vi "Array Of Variants To Class Types.vi"(7 "Elements":variant[](array[variant]), 8 "error in (no error)":errorcluster, 10 "Class types":variant[](array[variant]), 11 "Registry Variant Accessor in":refnum<class "CConfig Variant Accessor.lvclass">) -> (0 "error out":errorcluster, 2 "Class types":variant[](array[variant]), 3 "Registry Variant Accessor out":refnum<class "CConfig Variant Accessor.lvclass">)   [LabVIEW 2013, in "CConfig Variant Accessor.lvclass"]
doc: "Copyright 2018, Carya Automatisering, Wiebe Walstra."
uses:
  CConfig Variant Accessor.lvclass
  <vilib>/Utility/VariantDataType/Type.ctl
  <vilib>/Utility/VariantDataType/VariantType.lvlib
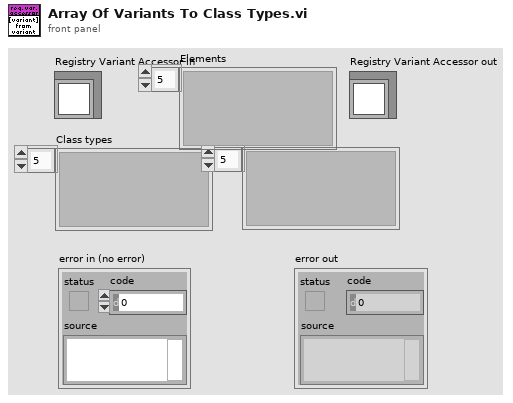
[diagram p1: front panel]
types:
  T1 = typedef "VariantType.lvlib/Type.ctl" = enum8{"Invalid Type", "Void", "I8", "I16", "I32", "I64", "U8", "U16", "U32", "U64", "Single Float", "Double Float", "Extended Float", "Single Complex", "Double Complex", "Extended Complex", "Enum U8", "Enum U16", "Enum U32", "Enum U64", "Single Float With Unit", "Double Float With Unit", "Extended Float With Unit", "Single Complex with Unit", "Double Complex with Unit", "Extended Complex with Unit", "Boolean", "String", "Path", "Picture", "Tag", "Array", "Cluster", "Variant", "LV Variant", "Waveform", "Timestamp", "Digital Waveform", "Digital Data", "ExpressData", "Refnum", "External Data", "VI", "Poly VI", "LabVIEW Class Instance", "Fixed Point"}
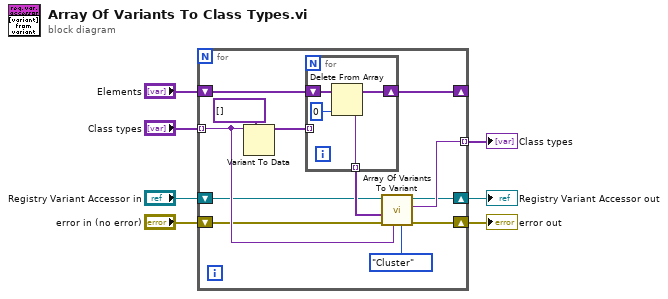
[diagram p0: block diagram]
diagram:
  n1 = for {
    tunnel: "Class types" -> [w14] mode=indexing
    shift-right: [w16] -> _
    shift-left: "Elements" -> [w17]
    tunnel: [w12] -> w1 mode=indexing
    shift-right: [w10] -> w3
    shift-left: "Registry Variant Accessor in" -> [w11]
    shift-right: [w8] -> w4
    shift-left: "error in (no error)" -> [w9]
    n2 = Variant To Data(type=variant[] [], Variant=w14) -> (data=w18:variant[])  [unwired: 1 in, 1 out]
    n3 = for {
      tunnel: w18 -> [_] mode=indexing
      shift-right: [w22] -> w16
      shift-left: w17 -> [w23]
      tunnel: [w20] -> w15 mode=indexing
      n4 = Delete From Array(array=w23, index=0) -> (deleted portion=w20:variant, array with subset deleted=w22:variant[])  [unwired: 1 in]
    }
    n5 = call-dynamic "Array Of Variants To Variant.vi"("Type Enum [auto]"=Type."Cluster", "Variant"=w14, "error in (no error)"=w9, "Elements"=w15, "Registry Variant Accessor in"=w11) -> ("error out"=w8:errorcluster, "Variant"=w12:variant, "Registry Variant Accessor out"=w10:refnum<class "CConfig Variant Accessor.lvclass">)  [unwired: 4 in]
  }
  "error out" <- w4
  "Registry Variant Accessor out" <- w3
  "Class types" <- w1
